vi "Rendezvous global.vi"() -> ()   [LabVIEW 2017]
panel:
  in  "Number of acq. devs.":i32=1
  in  "Rendezvous":T1
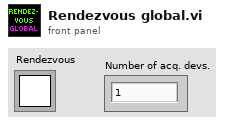
[diagram p1: front panel]
types:
  T1 = typedef "Rendezvous RefNum" = refnum<k1>
diagram:
